vi "Handle Error.vi"(8 "error in (no error)":errorcluster, 11 "Main in":refnum<class "Main.lvclass">) -> (0 "error out":errorcluster, 2 "stop actor?":bool=TRUE, 3 "Main out":refnum<class "Main.lvclass">)   [LabVIEW 2023, in "GUI.lvlib" / "Main.lvlib" / "Main.lvclass"]
doc: "(<B>Filename</B>: Actor Framework.lvlib:Actor.lvclass:Handle Error.vi)\n\nDefines how the actor handles an error that occurred while processing a message. By default, this method does nothing except stop the actor."
uses:
  Main.lvclass
  <vilib>/ActorFramework/Actor/Actor.lvclass
  GUI.lvlib
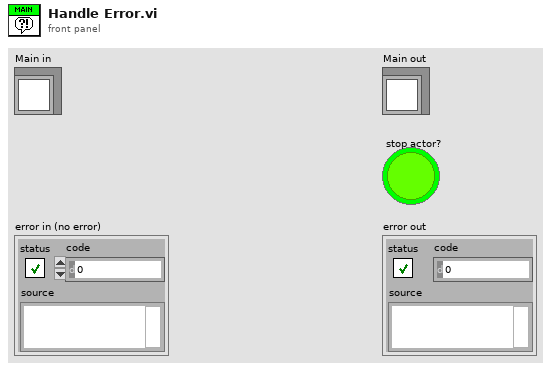
[diagram p1: front panel]
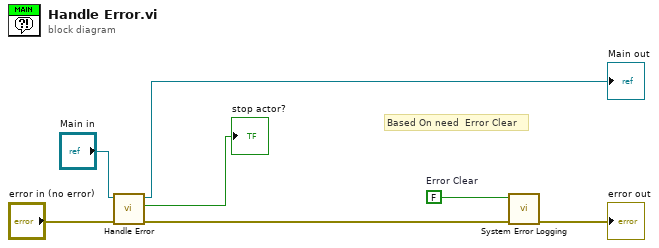
[diagram p0: block diagram]
diagram:
  w1 = FALSE  # Error Clear
  # "Based On need  Error Clear"
  n1 = call-parent "Handle Error.vi"("error in (no error)"="error in (no error)", "Actor in"="Main in") -> ("error out"=w3:errorcluster, "stop actor?"=→"stop actor?":bool, "Actor out"=→"Main out":refnum<class "Main.lvclass">)  [unwired: 7 in]
  n2 = call "System Error Logging.vi"("error in"=w3, "Error Clear"=w1) -> ("error out"=→"error out":errorcluster)  [unwired: 9 in]
